vi "Common Path String to Specific Windows Platform Path.vi"(4 "common path":string) -> (1 "specific path":path)   [LabVIEW 2020]
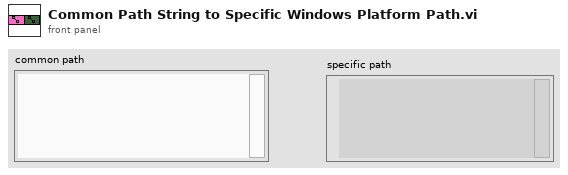
[diagram p1: front panel]
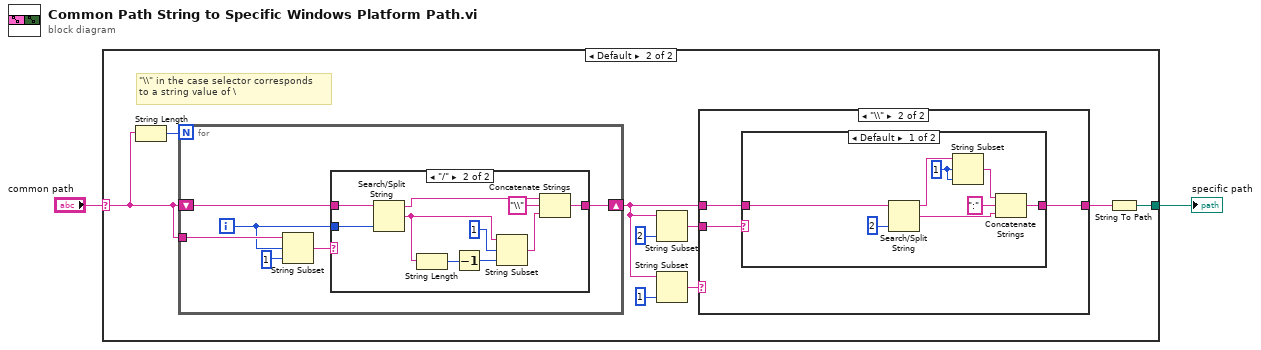
[diagram p0: block diagram]
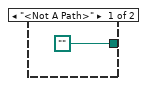
[diagram p2: hidden frame]
diagram:
  n1 = case shown="Default" "common path" {
    selector: "common path" -> [_ w4]
    tunnel: [path "" ("Not A Path Constant") w5] -> w2
    frame "<Not A Path>" {
    }
    frame Default {
      # "\"\\\\\" in the case selector corresponds\nto a string value of \\"
      n2 = String Length(string=w4) -> (length=w9:i32)
      n3 = for {
        N: w9 -> [_]
        tunnel: w4 -> [w16]
        shift-right: [w17] -> w10
        shift-left: w4 -> [w18]
        i -> [w15]
        n4 = String Subset(string=w16, offset (0)=w15, length (rest)=1 ("length")) -> (substring=w13:string)
        n5 = case shown="\"/\"" w13 {
          tunnel: w18 -> [w19 w29]
          tunnel: w15 -> [_ w21]
          tunnel: [w19 w27] -> w17
          frame Default {
          }
          frame "/" {
            n6 = Search/Split String(string=w29, offset (0)=w21) -> (substring before match=w28:string, match + rest of string=w25:string)  [unwired: 2 out]
            n7 = String Length(string=w25) -> (length=w24:i32)
            n8 = Decrement(x=w24) -> (x-1=w23:i32)
            n9 = String Subset(string=w25, offset (0)=1, length (rest)=w23) -> (substring=w20:string)
            n10 = Concatenate Strings(w28, "\\" ("x"), w20) -> (w27:string)
          }
        }
      }
      n11 = String Subset(string=w10, length (rest)=2 ("length")) -> (substring=w12:string)  [unwired: 1 out]
      n12 = String Subset(string=w10, length (rest)=1 ("length")) -> (substring=w11:string)  [unwired: 1 out]
      n13 = case shown="\"\\\\\"" w11 {
        tunnel: w10 -> [w30 w33]
        tunnel: [w30 w32] -> w7
        tunnel: w12 -> [_ w31]
        frame Default {
        }
        frame "\\" {
          n14 = case shown="Default" w31 {
            tunnel: w33 -> [w41 w42]
            tunnel: [w35 w42] -> w32
            frame Default {
              w34 = 1 ("offset (0)")
              n15 = Search/Split String(string=w41, offset (0)=2) -> (substring before match=w39:string, match + rest of string=w36:string)  [unwired: 2 out]
              n16 = String Subset(string=w39, offset (0)=w34, length (rest)=w34) -> (substring=w38:string)
              n17 = Concatenate Strings(w38, ":", w36) -> (w35:string)
            }
            frame "\\\\" {
              # "\"\\\\\\\\\" in the case selector corresponds\nto a string value of \\\\"
            }
          }
        }
      }
      n18 = String To Path(string=w7) -> (path=w5:path)
    }
  }
  "specific path" <- w2
